vi "circle+rectangle.vi"() -> ()   [LabVIEW 2017]
uses:
  <vilib>/Simulation/Scripting/Companion Diagram/SimConfigNode/SimParams.ctl
  <vilib>/Simulation/Scripting/Companion Diagram/SimConfigNode/_simSolvers.ctl
  <vilib>/Simulation/Implementation/Shared/SIMSCR Execution Mode.ctl
  <vilib>/Simulation/Param Hierarchy/Typedefs/SIMPH Param Control Actions.ctl
  <vilib>/Simulation/Implementation/Shared/NILVSim_ParamChanged.vi
  <vilib>/Simulation/Implementation/Shared/NILVSIM_BeginStep.vi
  <vilib>/Simulation/Implementation/Shared/NILVSim_Manager.vi
  <vilib>/Utility/error.llb/Clear Errors.vi
  <vilib>/Simulation/Implementation/Shared/NILVSim_FinalizeModel.vi
  <vilib>/DAQmx/read.llb/DAQmx Read (Counter DBL 1Chan 1Samp).vi
  <vilib>/DAQmx/read.llb/DAQmx Read (Digital Bool 1Line 1Point).vi
  917b7e52-755f-4d44-bea8-9e7c9beac24e.vi
  a58f9967-76f1-4ebc-ad3d-26e75a3ca160.vi
  <vilib>/DAQmx/write.llb/DAQmx Write (Analog DBL 1Chan 1Samp).vi
  <vilib>/DAQmx/create/channels.llb/DAQmx Create Channel (AO-Voltage-Basic).vi
  <vilib>/DAQmx/create/channels.llb/DAQmx Create Channel (DI-Digital Input).vi
  <vilib>/DAQmx/create/channels.llb/DAQmx Create Channel (CI-Count Edges).vi
  <vilib>/Simulation/Implementation/Shared/SIM Unbundle Sim Info.vi
  <vilib>/Simulation/Implementation/Shared/NILVSim_Initialize.vi
  <vilib>/Simulation/Utility/Implementation/NILVSim Get Time and IsAcceptedStep.vi
  <vilib>/Simulation/Implementation/Shared/SIMSH Read Queue.vi
  <vilib>/Simulation/Implementation/Shared/NILVSim_GetModelError.vi
  <vilib>/Simulation/Implementation/Shared/SIM Bundle Sim Info.vi
  <vilib>/DAQmx/miscellaneous.llb/DAQmx Fill In Error Info.vi
  <vilib>/Simulation/Implementation/XNodeFramework/SimXNode/SimX.xnode
  <vilib>/Simulation/Model Libraries/PID/SIM PID (Parallel).vi
  <vilib>/Simulation/Model Libraries/PID/SIM PID.vi
  <vilib>/Simulation/Scripting/Companion Diagram/SimConfigNode/SimDog.xnode
  <vilib>/Simulation/Model Libraries/PID/SIM PID (Academic).vi
  <vilib>/Simulation/Implementation/Shared/NI_SIM_Implementation.lvlib
panel:
  out "Boolean 2":bool
  out "reset":bool
  in  "checking re":bool
  in  "checking enums":T1(ring)
  in  "rectangle":bool
  in  "Boolean":bool
  in  "stage rectangle":T2(ring)
  out "Step 2I":bool
  out "Step 2G":bool
  out "Step 2E":bool
  out "stay1":dbl
  out "stay":dbl
  out "calculating error x":dbl
  out "calculating error y":dbl
  in  "origin":bool
  out "Previous Y":dbl
  out "Previous X":dbl
  out "Current Y":dbl
  out "Current X":dbl
  out "previous index":dbl
  out "both/reset enter":bool
  out "reset complete":bool
  out "x circle":bool
  out "y circle":bool
  out "Point circle is drawing":dbl
  out "false":bool
  in  "Radius 2":dbl
  out "No of Points":dbl
  out "Passing Y":dbl
  out "Y array":dbl[](array[numeric])
  out "array Y length 2":dbl
  out "Passing X":dbl
  out "X array":dbl[](array[numeric])
  out "array x Length 2":dbl
  in  "stage circle":T3(ring)
  in  "check instruc":bool
  out "x entered":dbl
  out "y enetred":dbl
  out "greater -1 x":bool
  out "less 1 x":bool
  out "direction selected":dbl
  out "at 2f":bool
  out "Step 2J":bool
  out "Step 2H":bool
  out "Shape drawing steps":enum16{"corner", "1st switch", "reverse"}(ring)
  out "Step 2D":bool
  out "c":bool
  in  "height":dbl
  in  "length":dbl
  in  "part":T4(ring)=enum."a"
  in  "Has encoders been reset?":enum16{"don't reset", "reset"}(ring)
  out "x distance currently being travelled":dbl
  out "y distance currently being travelled":dbl
  out "error calced":dbl
  out "p1 dis 2":dbl
  out "p1 dis":dbl
  out "error y":dbl
  out "calc distance y":dbl
  out "calc distanc x":dbl
  out "error x":dbl
  out "reached y":bool
  out "reached x":bool
  out "Numeric":dbl
  in  "Draw rectangle":bool
  in  "Draw circle":bool
  out "In drawing mode":bool
  in  "Right-Down":bool
  in  "Left-Up":bool
  in  "Left-Down":bool
  in  "Right-Up":bool
  in  "right":bool
  in  "left":bool
  in  "motor 2":dbl(slide)=1.5 scale=-10.0..10.0
  in  "down":bool
  in  "up":bool
  in  "Y Length":dbl=30.0
  in  "X Length":dbl=30.0
  in  "Motor 2 encoder":tag="Dev1/ctr1"
  out "Pulses M2":dbl format="%.2f"
  in  "Motor 1 encoder":tag="Dev1/ctr0"
  out "Pulses M1":dbl format="%.2f"
  out "Right":bool
  out "Bottom":bool
  out "Left":bool
  out "Top":bool
  in  "Switch 4/Line 3":tag="Dev1/port0/line3"
  in  "Switch 3/Line 2":tag="Dev1/port0/line2"
  in  "Switch 2/Line 1":tag="Dev1/port0/line1"
  in  "Switch 1/Line 0":tag="Dev1/port0/line0"
  in  "Motor stop":bool
  in  "Motor 1":tag="Dev1/ao0"
  in  "max Voltage":dbl=10.0
  in  "Min Voltage":dbl=-10.0
  in  "Motor 2":tag="Dev1/ao1"
  in  "motor 1":dbl(slide)=1.5 scale=-10.0..10.0
  in  "stop":bool
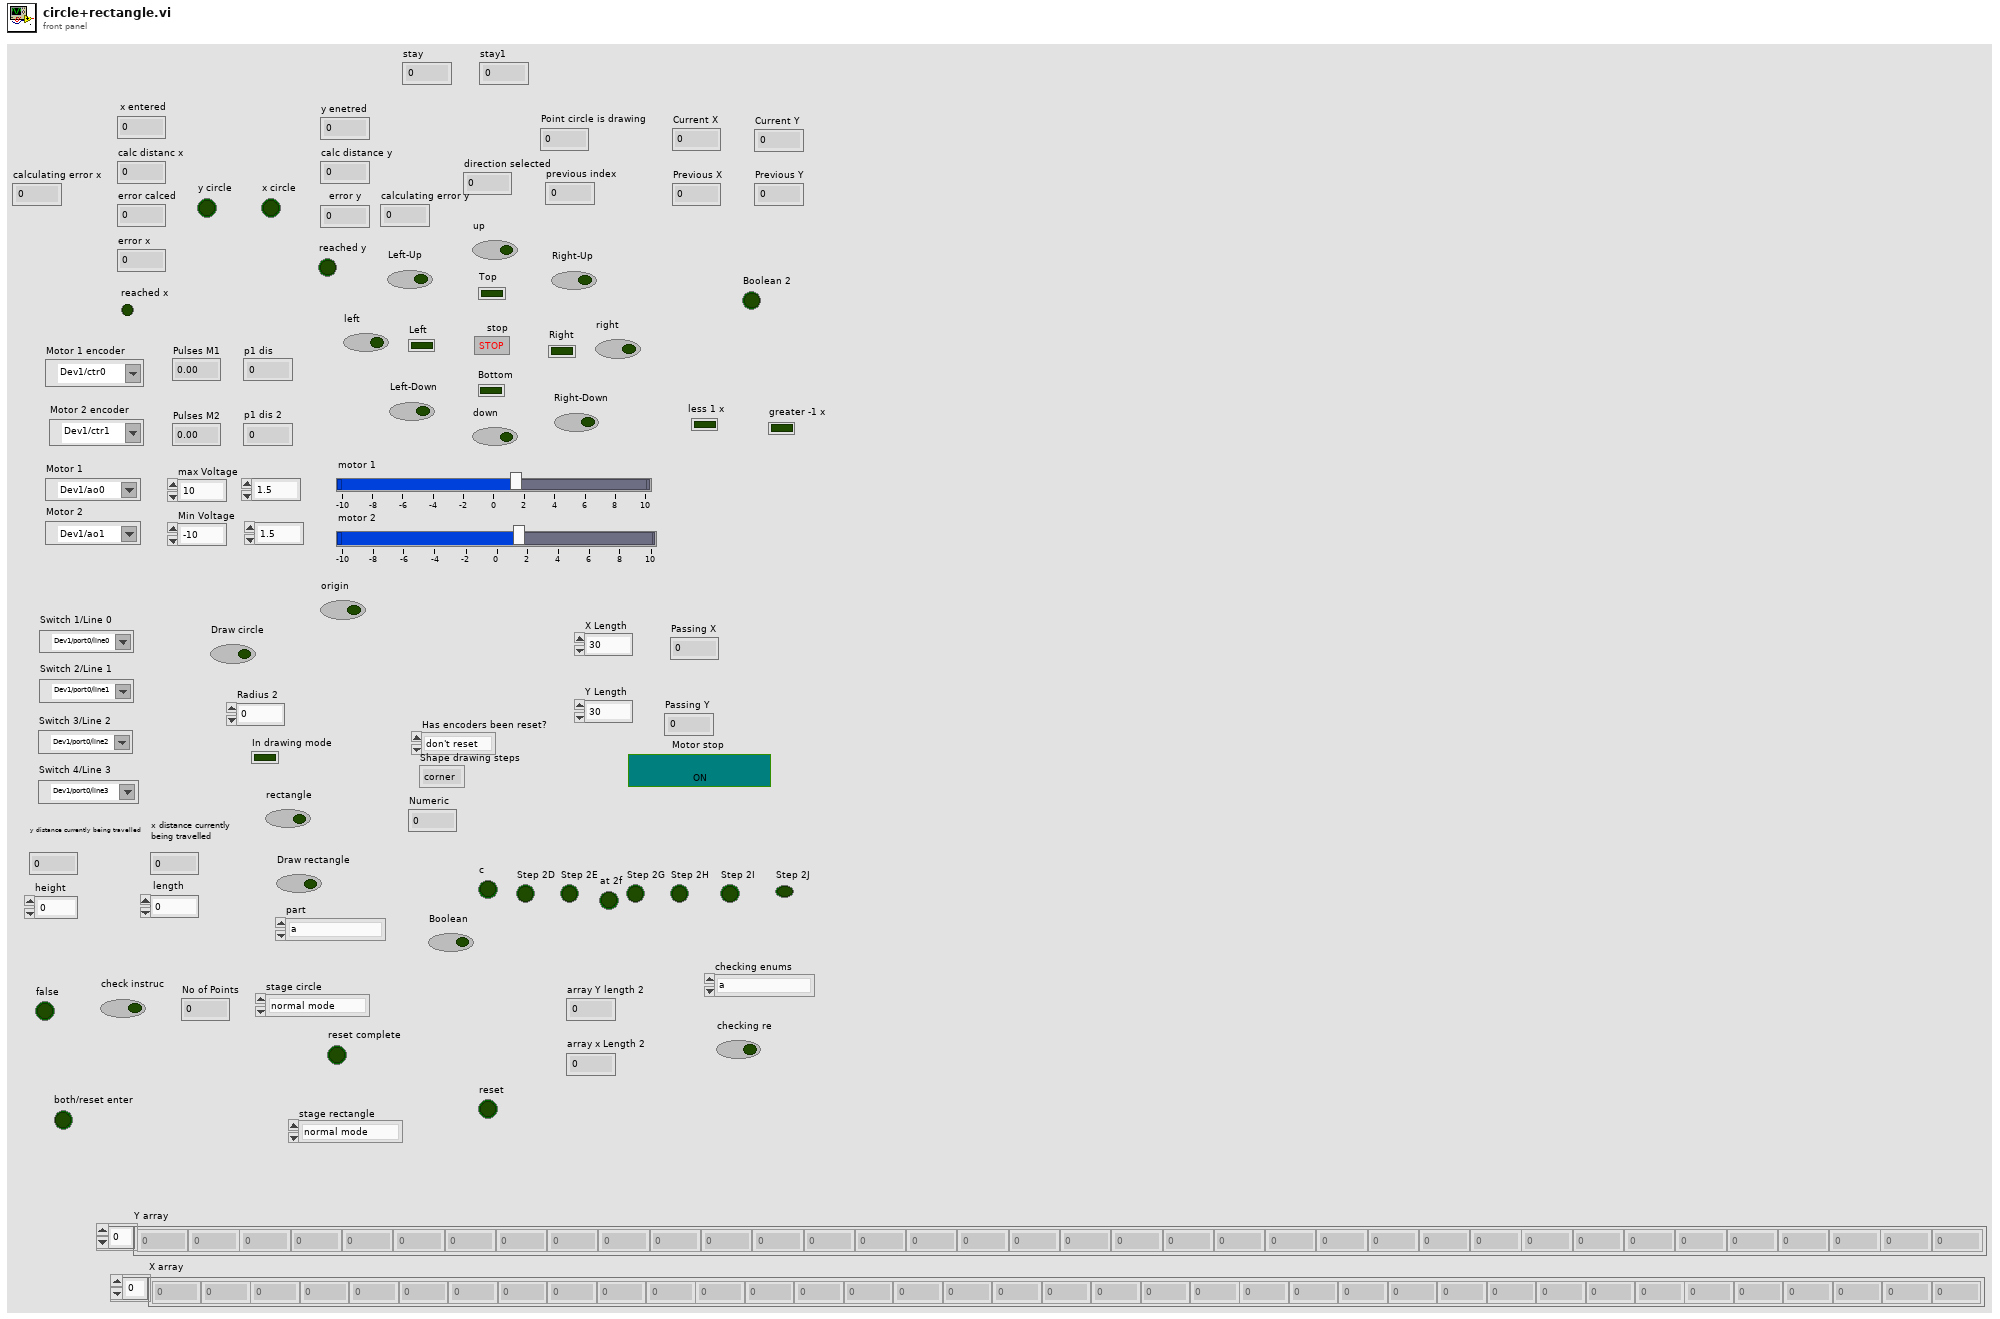
[diagram p1: front panel]
types:
  T1 = enum16{"a", "starting pt", "reset", "going right", "reset before down", "going down", "reset before left", "going left", "reset before up", "going up", "nothing"}
  T2 = enum16{"normal mode", "take to origin", "reset before start", "reset before right", "giving values right", "drawing right", "reset before down", "giving values down", "drawing down", "reset before left", "giving value left", "drawing left", "reset before up", "giving values up", "drawing up", "last step"}
  T3 = enum16{"normal mode", "take to origin", "reset before start", "create points", "draw points", "checking if draw", "reset draw counter"}
  T4 = enum16{"nothing", "j", "i", "h", "g", "f", "e", "d", "c", "b", "a"}
  T5 = enum16{"a", "starting pt", "reset", "going right", "reset before down", "going down", "reset before left", "going left", "reset before up", "going up"}
  T6 = enum16{"Simulate to Completion", "Single Time-Step Simulation (Fixed Step Only)"}
  T7 = typedef "SIMSCR Execution Mode.ctl" = enum16{"Simulate to Completion", "Single Time-Step Simulation (Fixed Step Only)"}
  T8 = typedef "SIMPH Param Control Actions.ctl" = enum16{"get params", "set params"}
  T9 = cluster{"SIMSH Sim Time":dbl, "SIM PID Derivative Gain.vi":cluster{"output":dbl}, "SIM PID Derivative Gain.vi - SIMSH":cluster{"SIMSH Sim Time":dbl, "t 3":dbl, "Select 2":cluster{"s? t:f":dbl}, "Equal?":cluster{"x = y?":bool}, "Or":cluster{"x .or. y?":bool}, "Equal To 0?":cluster{"x = 0?":bool}}, "High Frequency [s] (Tf)":dbl, "Gain":cluster{"output":dbl}, "Summation":cluster{"Result":dbl}, "Integral Gain - series.vi":cluster{"output":dbl}, "Integral Gain - series.vi - SIMSH":cluster{"SIMSH Sim Time":dbl, "Select 2":cluster{"s? t:f":dbl}, "integral in gain?":bool, "Integrator":cluster{"output y(t)":dbl}, "Gain 2":cluster{"output":dbl}, "Select":cluster{"s? t:f":dbl}, "Equal To 0?":cluster{"x = 0?":bool}, "Reciprocal":cluster{"1/x":dbl}}}
  T10 = typedef "SimParams.ctl" = cluster{"Initial Time (s)":dbl, "Final Time (s)":dbl, "Step Size (s)":dbl, "ODE Solver":T11, "Minimum Step Size (s)":dbl, "Maximum Step Size (s)":dbl, "Relative Tolerance":dbl, "Absolute Tolerance":dbl, "Software Timing":bool, "Initial Step Size (s)":dbl, "Automatic Fixed Step Size?":bool, "Automatic Discrete Step Size?":bool, "Discrete Step Size (s)":dbl, "Calculate using Time Step":bool, "Solver Wired?":bool, "Prev.Frm.Expected End":u64, "Prev.Frm.Actual End":u64, "Prev.Frm.Finished Late?":bool, "Prev.Iter.Expected End":u64, "Prev.Iter.Actual End":u64, "Prev.Iter.Finished Late?":bool, "Expected Iteration Start":u64, "Actual Iteration Start":u64, "Expected Frame Start":u64, "Actual Frame Start":u64, "Source Name":string, "Name":string, "Period":i64, "Deadline":i64, "Offset":i64, "Start":i64, "Priority":i32, "Timeout":i32, "Processor":i32, "Mode":enum32{"No Change", "Process missed periods, maintain original phase", "Discard missed periods, maintain original phase", "Process missed periods, ignore original phase", "Discard missed periods, ignore original phase"}, "Wakeup reason":enum32{"Normal", "Aborted", "Asynchronous wakeup", "Timing source error", "Timed loop error", "Timeout"}, "Error":errorcluster, "Source Type":string, "Secondary Source Type":string, "Global End Time":u64, "Global Start Time":u64, "Full Solver Reset":bool, "Execution Mode":T7, "Nan/Inf Check":bool, "Custom Solver Library":string, "Solver Is Variable":bool, "custom solver name":string, "Signal Collection Decimation":u32}
  T11 = typedef "_simSolvers.ctl" = enum16{"Runge-Kutta 1 (Euler)", "Runge-Kutta 2", "Runge-Kutta 3", "Runge-Kutta 4", "Runge-Kutta 23 (variable)", "Runge-Kutta 45 (variable)", "BDF (variable)", "Adams-Moulton (variable)", "Rosenbrock (variable)", "Discrete States Only", "SDIRK 4 (variable)", "Radau 5 (variable)", "Radau 9 (variable)", "Radau 13 (variable)", "Radau [Variable Order] (variable)", "Gear's Method (variable)", "Linearizer", "State Query", "Trim Eval", "Custom Solver"}
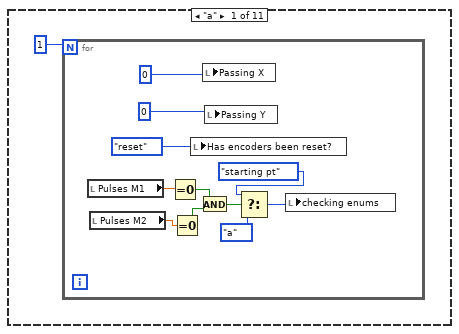
[diagram p3: hidden frame]
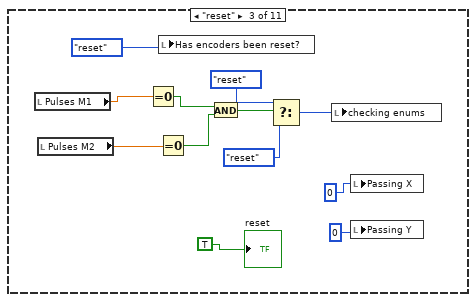
[diagram p4: hidden frame]
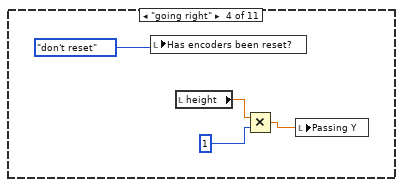
[diagram p5: hidden frame]
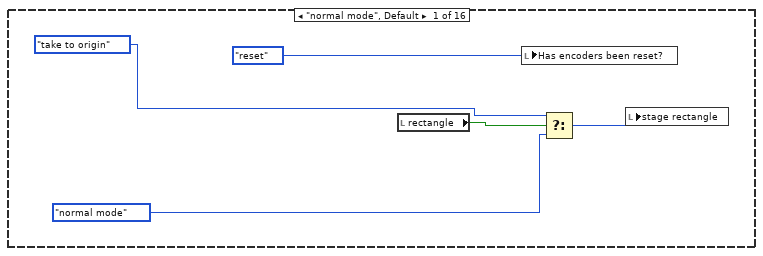
[diagram p14: hidden frame]
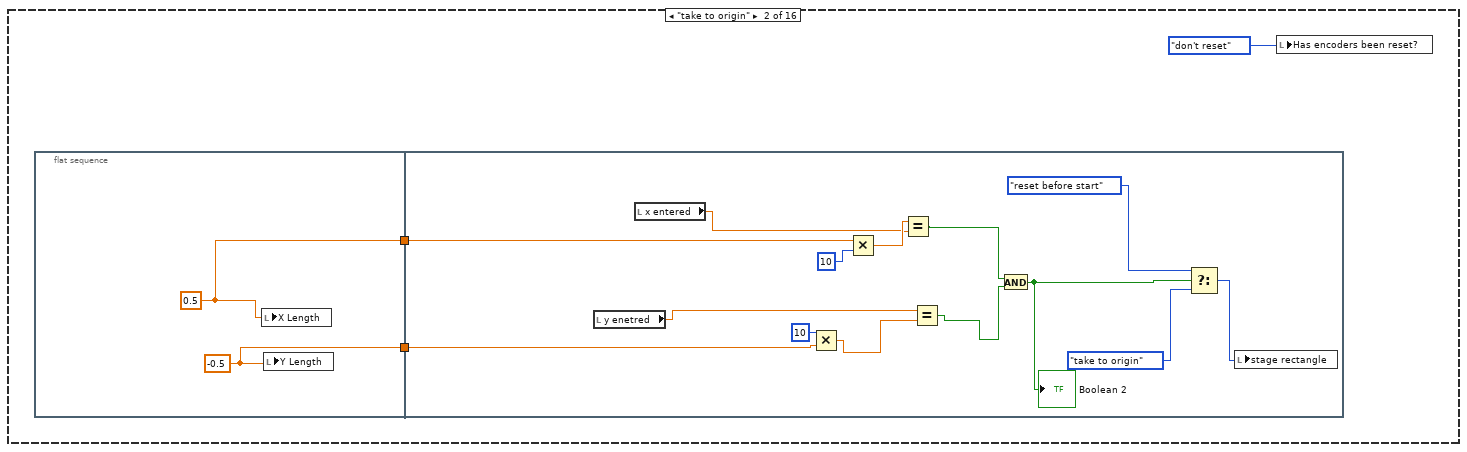
[diagram p15: hidden frame]
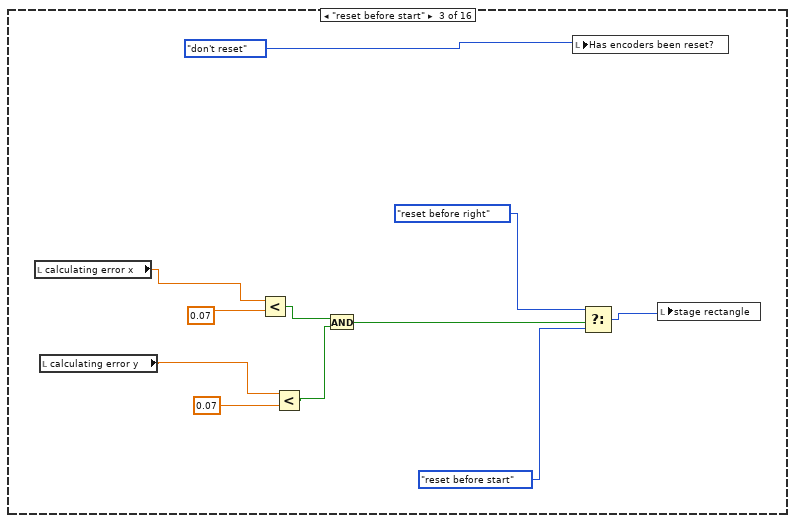
[diagram p16: hidden frame]
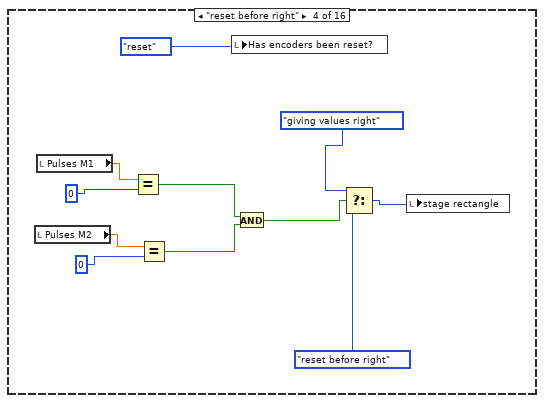
[diagram p17: hidden frame]
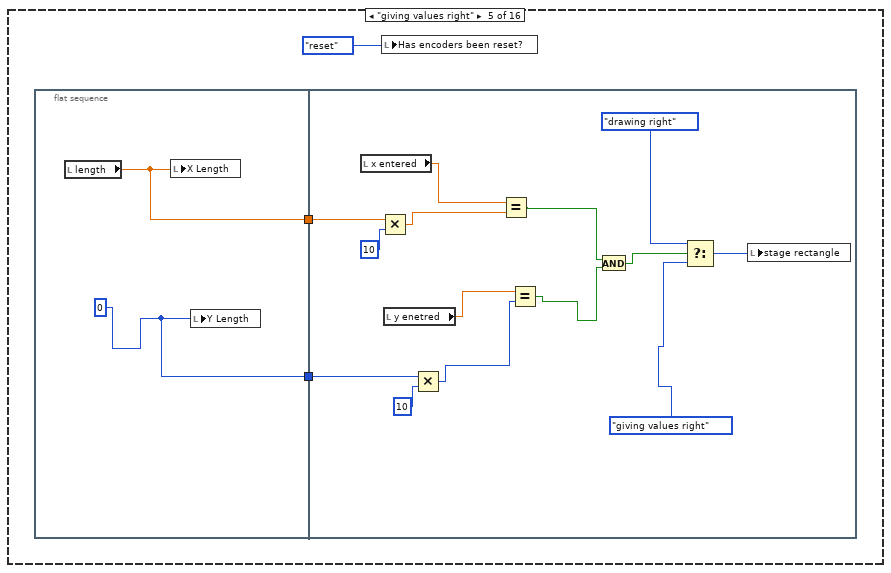
[diagram p18: hidden frame]
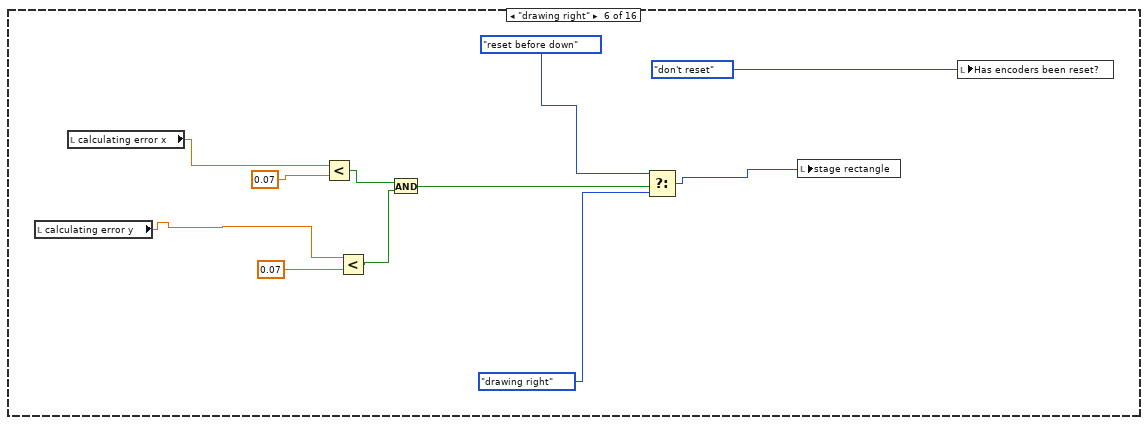
[diagram p19: hidden frame]
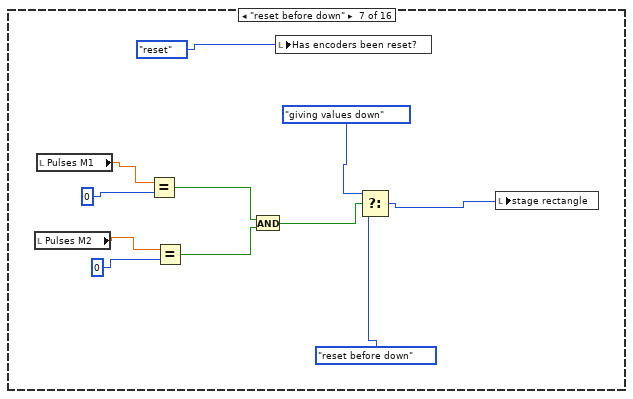
[diagram p20: hidden frame]
diagram:
  n1 = call-poly <vilib>:"DAQmx Create Virtual Channel.vi"("lines"="Switch 1/Line 0") -> ("task out"=w36:refnum<k21>, "error out"=w32:errorcluster)  [unwired: 13 in]
  n2 = call-poly <vilib>:"DAQmx Create Virtual Channel.vi"("lines"="Switch 2/Line 1") -> ("task out"=w35:refnum<k21>, "error out"=w31:errorcluster)  [unwired: 13 in]
  n3 = call-poly <vilib>:"DAQmx Create Virtual Channel.vi"("lines"="Switch 3/Line 2") -> ("task out"=w34:refnum<k21>, "error out"=w30:errorcluster)  [unwired: 13 in]
  n4 = call-poly <vilib>:"DAQmx Create Virtual Channel.vi"("lines"="Switch 4/Line 3") -> ("task out"=w33:refnum<k21>, "error out"=w29:errorcluster)  [unwired: 13 in]
  n5 = call-poly <vilib>:"DAQmx Create Virtual Channel.vi"("maximum value"="max Voltage", "minimum value"="Min Voltage", "physical channels"="Motor 1") -> ("task out"=w46:refnum<k21>, "error out"=w42:errorcluster)  [unwired: 11 in]
  n6 = call <vilib>:"DAQmx Start Task.vi"("task/channels in"=w36, "error in"=w32) -> ("task out"=w28:refnum<k21>, "error out"=w26:errorcluster)  [unwired: 12 in]
  n7 = call <vilib>:"DAQmx Start Task.vi"("task/channels in"=w35, "error in"=w31) -> ("task out"=w24:refnum<k21>, "error out"=w21:errorcluster)  [unwired: 12 in]
  n8 = call-poly <vilib>:"DAQmx Create Virtual Channel.vi"("maximum value"="max Voltage", "minimum value"="Min Voltage", "physical channels"="Motor 2") -> ("task out"=w49:refnum<k21>, "error out"=w41:errorcluster)  [unwired: 11 in]
  n9 = call-poly <vilib>:"DAQmx Create Virtual Channel.vi"("counter"="Motor 1 encoder") -> ("task out"=w7:refnum<k21>, "error out"=w2:errorcluster)  [unwired: 13 in]
  n10 = call-poly <vilib>:"DAQmx Create Virtual Channel.vi"("counter"="Motor 2 encoder") -> ("task out"=w6:refnum<k21>)  [unwired: 13 in, 1 out]
  n11 = call <vilib>:"DAQmx Start Task.vi"("task/channels in"=w34, "error in"=w30) -> ("task out"=w23:refnum<k21>, "error out"=w20:errorcluster)  [unwired: 12 in]
  n12 = call <vilib>:"DAQmx Start Task.vi"("task/channels in"=w33, "error in"=w29) -> ("task out"=w22:refnum<k21>, "error out"=w19:errorcluster)  [unwired: 12 in]
  n13 = call <vilib>:"DAQmx Start Task.vi"("task/channels in"=w7) -> ("task out"=w3:refnum<k21>)  [unwired: 13 in, 1 out]
  n14 = call <vilib>:"DAQmx Start Task.vi"("task/channels in"=w6) -> ("task out"=w1:refnum<k21>)  [unwired: 13 in, 1 out]
  n15 = while {
    tunnel: w49 -> [w240]
    tunnel: [w237] -> w48
    tunnel: w46 -> [w234]
    tunnel: [w233] -> w45
    tunnel: w42 -> [w231]
    tunnel: w41 -> [w230]
    tunnel: w28 -> [w224]
    tunnel: [w223] -> w27
    tunnel: w26 -> [w222]
    tunnel: [w221] -> w25
    tunnel: w24 -> [w220]
    tunnel: w23 -> [w219]
    tunnel: w22 -> [w218]
    tunnel: w21 -> [w217]
    tunnel: w20 -> [w216]
    tunnel: w19 -> [w215]
    tunnel: [w214] -> w18
    tunnel: [w213] -> w17
    tunnel: [w212] -> w16
    tunnel: [w211] -> w15
    tunnel: [w210] -> w14
    tunnel: [w209] -> w13
    tunnel: [w145] -> w10
    tunnel: w3 -> [w147]
    tunnel: w2 -> [w146]
    tunnel: w1 -> [w143]
    stop <- "stop" stop-if-true
    n16 = case shown="True" "check instruc" {
      frame False {
        "false" <- TRUE
      }
      frame True {
        n17 = case shown="\"reset before start\"" "stage circle" {
          frame "normal mode", Default {
            n18 = local read "check instruc"() -> (w613:bool)
            n19 = local write "Y Length"(0) -> ()
            n20 = local write "X Length"(0) -> ()
            n21 = local write "Has encoders been reset?"(enum16{"don't reset", "reset"}."reset") -> ()
            n22 = Select(t=T3."take to origin", s=w613, f=T3."normal mode") -> (s? t:f=w614:T3)
            n23 = local write "stage circle"(w614) -> ()
          }
          frame "take to origin" {
            n24 = flat-sequence {
              tunnel: [w621] -> w618
              tunnel: [w620] -> w617
              tunnel: w618 -> [w624]
              tunnel: w617 -> [w623]
              frame #0 {
                w620 = -1
                w621 = -1
                n25 = local write "X Length"(w621) -> ()
                n26 = local write "Y Length"(w620) -> ()
              }
              frame #1 {
                n27 = Multiply(x=10, y=w623) -> (x*y=w634:i32)
                n28 = local read "y enetred"() -> (w628:dbl)
                n29 = local read "x entered"() -> (w627:dbl)
                n30 = Multiply(x=10, y=w624) -> (x*y=w633:i32)
                n31 = Equal?(x=w627, y=w633) -> (x = y?=w630:bool)
                n32 = Equal?(x=w634, y=w628) -> (x = y?=w629:bool)
                n33 = And(x=w630, y=w629) -> (x .and. y?=w635:bool)
                n34 = Select(t=T3."reset before start", s=w635, f=T3."take to origin") -> (s? t:f=w622:T3)
                n35 = local write "stage circle"(w622) -> ()
              }
            }
            n36 = local write "Has encoders been reset?"(enum16{"don't reset", "reset"}."reset") -> ()
          }
          frame "reset before start" {
            n37 = local read "calculating error x"() -> (w645:dbl)
            n38 = local read "calculating error y"() -> (w643:dbl)
            n39 = Less?(x=w645, y=0.07) -> (x < y?=w641:bool)
            n40 = Less?(x=w643, y=0.07) -> (x < y?=w640:bool)
            n41 = local write "Has encoders been reset?"(enum16{"don't reset", "reset"}."don't reset") -> ()
            n42 = And(x=w641, y=w640) -> (x .and. y?=w639:bool)
            n43 = Select(t=T3."create points", s=w639, f=T3."reset before start") -> (s? t:f=w636:T3)
            n44 = local write "stage circle"(w636) -> ()
          }
          frame "create points" {
            n45 = for {
              N: 88 -> [_]
              shift-right: [w663] -> w654
              shift-left: _ -> [_]
              tunnel: [w663] -> w659 mode=indexing
              shift-right: [w662] -> w656
              shift-left: _ -> [_]
              tunnel: [w662] -> w658 mode=indexing
              i -> [w664]
              n46 = Multiply(x=2, y=3.141592653589793) -> (x*y=w667:dbl)
              n47 = Increment(x=w664) -> (x+1=w665:i32)
              n48 = Divide(x=w667, y=88) -> (x/y=w669:dbl)
              n49 = Multiply(x=w669, y=w665) -> (x*y=w666:dbl)
              n50 = Cosine(x=w666) -> (cos(x)=w672:dbl)
              n51 = Sine(x=w666) -> (sin(x)=w673:dbl)
              n52 = Multiply(x=w673, y="Radius 2") -> (x*y=w663:dbl)
              n53 = Multiply(x=w672, y="Radius 2") -> (x*y=w662:dbl)
              "No of Points" <- w664
            }
            "Passing Y" <- w654
            "Y array" <- w659
            "Passing X" <- w656
            "X array" <- w658
            n54 = local read "No of Points"() -> (w653:dbl)
            n55 = Equal?(x=w653, y=87) -> (x = y?=w650:bool)
            n56 = local write "Has encoders been reset?"(enum16{"don't reset", "reset"}."don't reset") -> ()
            n57 = Select(t=T3."draw points", s=w650, f=T3."create points") -> (s? t:f=w660:T3)
            n58 = local write "stage circle"(w660) -> ()
            n59 = Array Size(array=w659) -> (size(s)=→"array Y length 2":i32)
            n60 = Array Size(array=w658) -> (size(s)=→"array x Length 2":i32)
          }
          frame "draw points" {
            n61 = flat-sequence {
              frame #0 {
                n62 = local read "Point circle is drawing"() -> (w702:dbl)
                n63 = local read "previous index"() -> (w694:dbl)
                n64 = local read "Y array"() -> (w695:dbl[])
                n65 = local read "X array"() -> (w696:dbl[])
                n66 = Index Array(array=w695, index=w694) -> (element=→"Previous Y":dbl)
                n67 = Index Array(array=w696, index=w694) -> (element=→"Previous X":dbl)
                n68 = local read "X array"() -> (w697:dbl[])
                n69 = local read "Previous X"() -> (w684:dbl)
                n70 = local read "Current X"() -> (w689:dbl)
                n71 = local read "Y array"() -> (w698:dbl[])
                n72 = local read "Current X"() -> (w687:dbl)
                n73 = Greater Or Equal?(x=w702, y=89) -> (x >= y?=w700:bool)
                n74 = Not Equal To 0?(x=w702) -> (x != 0?=w690:bool)
                n75 = local read "Previous Y"() -> (w685:dbl)
                n76 = local read "Current Y"() -> (w686:dbl)
                n77 = Index Array(array=w697, index=w702) -> (element=→"Current X":dbl)
                n78 = Subtract(x=w687, y=w684) -> (x-y=w682:dbl)
                n79 = Select(t=w682, s=w690, f=w689) -> (s? t:f=w679:dbl)
                n80 = Select(t=T3."normal mode", s=w700, f=T3."draw points") -> (s? t:f=w699:T3)
                n81 = Index Array(array=w698, index=w702) -> (element=→"Current Y":dbl)
                n82 = Subtract(x=w686, y=w685) -> (x-y=w681:dbl)
                n83 = local read "Current Y"() -> (w688:dbl)
                n84 = local write "X Length"(w679) -> ()
                n85 = Not(x=w700) -> (.not. x?=w701:bool)
                n86 = local write "stage circle"(w699) -> ()
                n87 = Not Equal To 0?(x=w702) -> (x != 0?=w691:bool)
                n88 = Select(t=w681, s=w691, f=w688) -> (s? t:f=w680:dbl)
                n89 = local write "Y Length"(w680) -> ()
                n90 = local write "check instruc"(w701) -> ()
              }
              frame #1 {
                n91 = local write "stage circle"(T3."checking if draw") -> ()
              }
            }
            n92 = local write "Has encoders been reset?"(enum16{"don't reset", "reset"}."don't reset") -> ()
          }
          frame "checking if draw" {
            n93 = local read "calculating error x"() -> (w707:dbl)
            n94 = local read "calculating error y"() -> (w705:dbl)
            n95 = local read "Point circle is drawing"() -> (w710:dbl)
            n96 = Greater Or Equal?(x=0.07, y=w707) -> (x >= y?=w713:bool)
            "x circle" <- w713
            n97 = Greater Or Equal?(x=0.07, y=w705) -> (x >= y?=w714:bool)
            "y circle" <- w714
            n98 = And(x=w714, y=w713) -> (x .and. y?=w711:bool)
            "both/reset enter" <- w711
            n99 = Increment(x=w710) -> (x+1=w716:dbl)
            n100 = Select(t=w716, s=w711, f=w710) -> (s? t:f=→"Point circle is drawing":dbl)
            n101 = Select(t=T3."reset draw counter", s=w711, f=T3."checking if draw") -> (s? t:f=w712:T3)
            n102 = local write "stage circle"(w712) -> ()
          }
          frame "reset draw counter" {
            n103 = for {
              N: 1 -> [_]
              i -> [w721]
              n104 = local read "Point circle is drawing"() -> (w726:dbl)
              n105 = local read "Pulses M2"() -> (w731:dbl)
              n106 = local read "Pulses M1"() -> (w732:dbl)
              n107 = Equal To 0?(x=w731) -> (x = 0?=w730:bool)
              n108 = Equal To 0?(x=w732) -> (x = 0?=w728:bool)
              n109 = local read "previous index"() -> (w723:dbl)
              n110 = local write "Has encoders been reset?"(enum16{"don't reset", "reset"}."reset") -> ()
              n111 = And(x=w728, y=w730) -> (x .and. y?=w729:bool)
              n112 = Subtract(x=w726, y=1) -> (x-y=w724:dbl)
              n113 = Select(t=T3."draw points", s=w729, f=T3."reset draw counter") -> (s? t:f=w733:T3)
              n114 = Equal To 0?(x=w721) -> (x = 0?=w720:bool)
              n115 = local write "stage circle"(w733) -> ()
              n116 = Select(t=w724, s=w720, f=w723) -> (s? t:f=→"previous index":dbl)
              "reset complete" <- TRUE
            }
          }
        }
      }
    }
    n117 = case shown="True" "rectangle" {
      frame False {
      }
      frame True {
        n118 = case shown="\"giving value left\"" "stage rectangle" {
          frame "normal mode", Default {
            n119 = local read "rectangle"() -> (w288:bool)
            n120 = local write "Has encoders been reset?"(enum16{"don't reset", "reset"}."reset") -> ()
            n121 = Select(t=T2."take to origin", s=w288, f=T2."normal mode") -> (s? t:f=w286:T2)
            n122 = local write "stage rectangle"(w286) -> ()
          }
          frame "take to origin" {
            n123 = flat-sequence {
              tunnel: [w293] -> w290
              tunnel: [w292] -> w289
              tunnel: w290 -> [w303]
              tunnel: w289 -> [w302]
              frame #0 {
                w293 = -0.5
                w292 = 0.5
                n124 = local write "X Length"(w292) -> ()
                n125 = local write "Y Length"(w293) -> ()
              }
              frame #1 {
                n126 = local read "y enetred"() -> (w297:dbl)
                n127 = local read "x entered"() -> (w298:dbl)
                n128 = Multiply(x=10, y=w303) -> (x*y=w305:dbl)
                n129 = Multiply(x=w302, y=10) -> (x*y=w301:dbl)
                n130 = Equal?(x=w301, y=w298) -> (x = y?=w300:bool)
                n131 = Equal?(x=w297, y=w305) -> (x = y?=w299:bool)
                n132 = And(x=w300, y=w299) -> (x .and. y?=w307:bool)
                "Boolean 2" <- w307
                n133 = Select(t=T2."reset before start", s=w307, f=T2."take to origin") -> (s? t:f=w296:T2)
                n134 = local write "stage rectangle"(w296) -> ()
              }
            }
            n135 = local write "Has encoders been reset?"(enum16{"don't reset", "reset"}."don't reset") -> ()
          }
          frame "reset before start" {
            n136 = local read "calculating error x"() -> (w312:dbl)
            n137 = local read "calculating error y"() -> (w311:dbl)
            n138 = Less?(x=w312, y=0.07) -> (x < y?=w313:bool)
            n139 = Less?(x=w311, y=0.07) -> (x < y?=w315:bool)
            n140 = And(x=w313, y=w315) -> (x .and. y?=w310:bool)
            n141 = local write "Has encoders been reset?"(enum16{"don't reset", "reset"}."don't reset") -> ()
            n142 = Select(t=T2."reset before right", s=w310, f=T2."reset before start") -> (s? t:f=w317:T2)
            n143 = local write "stage rectangle"(w317) -> ()
          }
          frame "reset before right" {
            n144 = local read "Pulses M2"() -> (w328:dbl)
            n145 = local read "Pulses M1"() -> (w329:dbl)
            n146 = Equal?(x=w329, y=0) -> (x = y?=w327:bool)
            n147 = Equal?(x=w328, y=0) -> (x = y?=w326:bool)
            n148 = local write "Has encoders been reset?"(enum16{"don't reset", "reset"}."reset") -> ()
            n149 = And(x=w327, y=w326) -> (x .and. y?=w325:bool)
            n150 = Select(t=T2."giving values right", s=w325, f=T2."reset before right") -> (s? t:f=w324:T2)
            n151 = local write "stage rectangle"(w324) -> ()
          }
          frame "giving values right" {
            n152 = flat-sequence {
              tunnel: [w333] -> w332
              tunnel: [w334] -> w331
              tunnel: w332 -> [w344]
              tunnel: w331 -> [w343]
              frame #0 {
                w333 = 0
                n153 = local read "length"() -> (w334:dbl)
                n154 = local write "X Length"(w334) -> ()
                n155 = local write "Y Length"(w333) -> ()
              }
              frame #1 {
                n156 = local read "x entered"() -> (w341:dbl)
                n157 = Multiply(x=w343, y=10) -> (x*y=w342:dbl)
                n158 = local read "y enetred"() -> (w339:dbl)
                n159 = Multiply(x=w344, y=10) -> (x*y=w340:i32)
                n160 = Equal?(x=w341, y=w342) -> (x = y?=w346:bool)
                n161 = Equal?(x=w339, y=w340) -> (x = y?=w345:bool)
                n162 = And(x=w346, y=w345) -> (x .and. y?=w337:bool)
                n163 = Select(t=T2."drawing right", s=w337, f=T2."giving values right") -> (s? t:f=w338:T2)
                n164 = local write "stage rectangle"(w338) -> ()
              }
            }
            n165 = local write "Has encoders been reset?"(enum16{"don't reset", "reset"}."reset") -> ()
          }
          frame "drawing right" {
            n166 = local read "calculating error y"() -> (w356:dbl)
            n167 = local read "calculating error x"() -> (w355:dbl)
            n168 = Less?(x=w355, y=0.07) -> (x < y?=w358:bool)
            n169 = Less?(x=w356, y=0.07) -> (x < y?=w359:bool)
            n170 = And(x=w358, y=w359) -> (x .and. y?=w357:bool)
            n171 = Select(t=T2."reset before down", s=w357, f=T2."drawing right") -> (s? t:f=w354:T2)
            n172 = local write "stage rectangle"(w354) -> ()
            n173 = local write "Has encoders been reset?"(enum16{"don't reset", "reset"}."don't reset") -> ()
          }
          frame "reset before down" {
            n174 = local read "Pulses M2"() -> (w364:dbl)
            n175 = local read "Pulses M1"() -> (w365:dbl)
            n176 = Equal?(x=w365, y=0) -> (x = y?=w370:bool)
            n177 = Equal?(x=w364, y=0) -> (x = y?=w369:bool)
            n178 = And(x=w370, y=w369) -> (x .and. y?=w368:bool)
            n179 = local write "Has encoders been reset?"(enum16{"don't reset", "reset"}."reset") -> ()
            n180 = Select(t=T2."giving values down", s=w368, f=T2."reset before down") -> (s? t:f=w361:T2)
            n181 = local write "stage rectangle"(w361) -> ()
          }
          frame "giving values down" {
            n182 = flat-sequence {
              tunnel: [w377] -> w373
              tunnel: [w374] -> w372
              tunnel: w373 -> [w382]
              tunnel: w372 -> [w381]
              frame #0 {
                w377 = 0
                n183 = local read "height"() -> (w376:dbl)
                n184 = Multiply(x=w376, y=-1) -> (x*y=w374:dbl)
                n185 = local write "X Length"(w377) -> ()
                n186 = local write "Y Length"(w374) -> ()
              }
              frame #1 {
                n187 = local read "y enetred"() -> (w383:dbl)
                n188 = local read "x entered"() -> (w384:dbl)
                n189 = Multiply(x=w382, y=10) -> (x*y=w390:i32)
                n190 = Multiply(x=w381, y=10) -> (x*y=w388:dbl)
                n191 = Equal?(x=w384, y=w390) -> (x = y?=w385:bool)
                n192 = Equal?(x=w383, y=w388) -> (x = y?=w386:bool)
                n193 = And(x=w385, y=w386) -> (x .and. y?=w387:bool)
                n194 = Select(t=T2."drawing down", s=w387, f=T2."giving values down") -> (s? t:f=w378:T2)
                n195 = local write "stage rectangle"(w378) -> ()
              }
            }
            n196 = local write "Has encoders been reset?"(enum16{"don't reset", "reset"}."reset") -> ()
          }
          frame "drawing down" {
            n197 = local read "calculating error y"() -> (w397:dbl)
            n198 = local read "calculating error x"() -> (w396:dbl)
            n199 = Less?(x=w396, y=0.07) -> (x < y?=w401:bool)
            n200 = Less?(x=w397, y=0.07) -> (x < y?=w402:bool)
            n201 = And(x=w401, y=w402) -> (x .and. y?=w400:bool)
            n202 = Select(t=T2."reset before left", s=w400, f=T2."drawing down") -> (s? t:f=w393:T2)
            n203 = local write "Has encoders been reset?"(enum16{"don't reset", "reset"}."don't reset") -> ()
            n204 = local write "stage rectangle"(w393) -> ()
          }
          frame "reset before left" {
            n205 = local read "Pulses M1"() -> (w409:dbl)
            n206 = local read "Pulses M2"() -> (w408:dbl)
            n207 = Equal?(x=w409, y=0) -> (x = y?=w413:bool)
            n208 = Equal?(x=w408, y=0) -> (x = y?=w412:bool)
            n209 = And(x=w413, y=w412) -> (x .and. y?=w407:bool)
            n210 = Select(t=T2."giving value left", s=w407, f=T2."reset before left") -> (s? t:f=w404:T2)
            n211 = local write "stage rectangle"(w404) -> ()
            n212 = local write "Has encoders been reset?"(enum16{"don't reset", "reset"}."reset") -> ()
          }
          frame "giving value left" {
            n213 = flat-sequence {
              tunnel: [w420] -> w416
              tunnel: [w417] -> w415
              tunnel: w416 -> [w430]
              tunnel: w415 -> [w429]
              frame #0 {
                w420 = 0
                n214 = local read "length"() -> (w418:dbl)
                n215 = Multiply(x=w418, y=-1) -> (x*y=w417:dbl)
                n216 = local write "X Length"(w417) -> ()
                n217 = local write "Y Length"(w420) -> ()
              }
              frame #1 {
                n218 = local read "x entered"() -> (w428:dbl)
                n219 = local read "y enetred"() -> (w427:dbl)
                n220 = Multiply(x=w429, y=10) -> (x*y=w433:dbl)
                n221 = Multiply(x=w430, y=10) -> (x*y=w431:i32)
                n222 = Equal?(x=w428, y=w433) -> (x = y?=w425:bool)
                n223 = Equal?(x=w427, y=w431) -> (x = y?=w424:bool)
                n224 = And(x=w425, y=w424) -> (x .and. y?=w426:bool)
                n225 = Select(t=T2."drawing left", s=w426, f=T2."giving value left") -> (s? t:f=w421:T2)
                n226 = local write "stage rectangle"(w421) -> ()
              }
            }
            n227 = local write "Has encoders been reset?"(enum16{"don't reset", "reset"}."reset") -> ()
          }
          frame "drawing left" {
            n228 = local read "calculating error x"() -> (w439:dbl)
            n229 = local read "calculating error y"() -> (w440:dbl)
            n230 = Less?(x=w439, y=0.07) -> (x < y?=w444:bool)
            n231 = Less?(x=w440, y=0.07) -> (x < y?=w445:bool)
            n232 = And(x=w444, y=w445) -> (x .and. y?=w443:bool)
            n233 = Select(t=T2."reset before up", s=w443, f=T2."drawing left") -> (s? t:f=w436:T2)
            n234 = local write "Has encoders been reset?"(enum16{"don't reset", "reset"}."don't reset") -> ()
            n235 = local write "stage rectangle"(w436) -> ()
          }
          frame "reset before up" {
            n236 = local read "Pulses M1"() -> (w451:dbl)
            n237 = local read "Pulses M2"() -> (w450:dbl)
            n238 = Equal?(x=w451, y=0) -> (x = y?=w456:bool)
            n239 = Equal?(x=w450, y=0) -> (x = y?=w455:bool)
            n240 = And(x=w456, y=w455) -> (x .and. y?=w452:bool)
            n241 = Select(t=T2."giving values up", s=w452, f=T2."reset before up") -> (s? t:f=w447:T2)
            n242 = local write "Has encoders been reset?"(enum16{"don't reset", "reset"}."reset") -> ()
            n243 = local write "stage rectangle"(w447) -> ()
          }
          frame "giving values up" {
            n244 = flat-sequence {
              tunnel: [w461] -> w459
              tunnel: [w460] -> w458
              tunnel: w459 -> [w471]
              tunnel: w458 -> [w470]
              frame #0 {
                w460 = 0
                n245 = local read "height"() -> (w461:dbl)
                n246 = local write "X Length"(w460) -> ()
                n247 = local write "Y Length"(w461) -> ()
              }
              frame #1 {
                n248 = local read "x entered"() -> (w473:dbl)
                n249 = local read "y enetred"() -> (w472:dbl)
                n250 = Multiply(x=w470, y=10) -> (x*y=w475:i32)
                n251 = Multiply(x=w471, y=10) -> (x*y=w474:dbl)
                n252 = Equal?(x=w473, y=w475) -> (x = y?=w468:bool)
                n253 = Equal?(x=w472, y=w474) -> (x = y?=w467:bool)
                n254 = And(x=w468, y=w467) -> (x .and. y?=w469:bool)
                n255 = Select(t=T2."drawing up", s=w469, f=T2."giving values up") -> (s? t:f=w464:T2)
                n256 = local write "stage rectangle"(w464) -> ()
              }
            }
            n257 = local write "Has encoders been reset?"(enum16{"don't reset", "reset"}."reset") -> ()
          }
          frame "drawing up" {
            n258 = local read "calculating error x"() -> (w481:dbl)
            n259 = local read "calculating error y"() -> (w480:dbl)
            n260 = Less?(x=w481, y=0.07) -> (x < y?=w485:bool)
            n261 = Less?(x=w480, y=0.07) -> (x < y?=w486:bool)
            n262 = And(x=w485, y=w486) -> (x .and. y?=w484:bool)
            n263 = Select(t=T2."last step", s=w484, f=T2."drawing up") -> (s? t:f=w477:T2)
            n264 = local write "Has encoders been reset?"(enum16{"don't reset", "reset"}."don't reset") -> ()
            n265 = local write "stage rectangle"(w477) -> ()
          }
          frame "last step" {
            n266 = local write "X Length"(0) -> ()
            n267 = local write "Y Length"(0) -> ()
            n268 = local write "Has encoders been reset?"(enum16{"don't reset", "reset"}."reset") -> ()
          }
        }
      }
    }
    n269 = case shown="True" "checking re" {
      frame False {
      }
      frame True {
        n270 = case shown="\"starting pt\"" "checking enums" {
          frame "a" {
            n271 = for {
              N: 1 -> [_]
              n272 = local read "Pulses M1"() -> (w250:dbl)
              n273 = local read "Pulses M2"() -> (w249:dbl)
              n274 = Equal To 0?(x=w250) -> (x = 0?=w248:bool)
              n275 = Equal To 0?(x=w249) -> (x = 0?=w243:bool)
              n276 = local write "Has encoders been reset?"(enum16{"don't reset", "reset"}."reset") -> ()
              n277 = And(x=w248, y=w243) -> (x .and. y?=w247:bool)
              n278 = local write "Passing X"(0) -> ()
              n279 = local write "Passing Y"(0) -> ()
              n280 = Select(t=T5."starting pt", s=w247, f=T5."a") -> (s? t:f=w244:T5)
              n281 = local write "checking enums"(w244) -> ()
            }
          }
          frame "starting pt" {
            n282 = flat-sequence {
              frame #0 {
                n283 = local write "Passing Y"(10) -> ()
                n284 = local write "Passing X"(-6) -> ()
              }
            }
            n285 = local read "calculating error x"() -> (w263:dbl)
            n286 = local read "calculating error y"() -> (w261:dbl)
            n287 = local write "Has encoders been reset?"(enum16{"don't reset", "reset"}."don't reset") -> ()
            n288 = Less?(x=w263, y=0.07) -> (x < y?=w258:bool)
            n289 = Less?(x=w261, y=0.07) -> (x < y?=w259:bool)
            n290 = And(x=w258, y=w259) -> (x .and. y?=w257:bool)
            n291 = Select(t=T5."reset", s=w257, f=T5."starting pt") -> (s? t:f=w254:T5)
            n292 = local write "checking enums"(w254) -> ()
          }
          frame "reset" {
            (unwired) 0
            n293 = local read "Pulses M1"() -> (w277:dbl)
            n294 = local read "Pulses M2"() -> (w276:dbl)
            n295 = Equal To 0?(x=w277) -> (x = 0?=w274:bool)
            n296 = Equal To 0?(x=w276) -> (x = 0?=w275:bool)
            n297 = local write "Has encoders been reset?"(enum16{"don't reset", "reset"}."reset") -> ()
            n298 = And(x=w274, y=w275) -> (x .and. y?=w273:bool)
            n299 = Select(t=T5."reset", s=w273, f=T5."reset") -> (s? t:f=w270:T5)
            n300 = local write "checking enums"(w270) -> ()
            n301 = local write "Passing X"(0) -> ()
            n302 = local write "Passing Y"(0) -> ()
            "reset" <- TRUE
          }
          frame "going right" {
            n303 = local write "Has encoders been reset?"(enum16{"don't reset", "reset"}."don't reset") -> ()
            n304 = local read "height"() -> (w280:dbl)
            n305 = Multiply(x=w280, y=1) -> (x*y=w281:dbl)
            n306 = local write "Passing Y"(w281) -> ()
          }
          frame "reset before down" {
          }
          frame "going down" {
          }
          frame "reset before left" {
          }
          frame "going left" {
          }
          frame "reset before up" {
          }
          frame "going up" {
          }
          frame "nothing" {
          }
        }
      }
    }
    n307 = case shown="True" "Boolean" {
      frame False {
      }
      frame True {
        n308 = case shown="\"d\"" "part" {
          frame "a" {
            n309 = for {
              N: 1 -> [_]
              n310 = local read "Pulses M1"() -> (w498:dbl)
              n311 = local read "Pulses M2"() -> (w497:dbl)
              n312 = Equal To 0?(x=w497) -> (x = 0?=w500:bool)
              n313 = Equal To 0?(x=w498) -> (x = 0?=w499:bool)
              n314 = local write "Has encoders been reset?"(enum16{"don't reset", "reset"}."reset") -> ()
              n315 = And(x=w499, y=w500) -> (x .and. y?=w492:bool)
              n316 = local write "Passing X"(0) -> ()
              n317 = local write "Passing Y"(0) -> ()
              n318 = Select(t=T4."b", s=w492, f=T4."a") -> (s? t:f=w495:T4)
              n319 = local write "part"(w495) -> ()
            }
          }
          frame "b" {
            n320 = local read "calculating error x"() -> (w511:dbl)
            n321 = local read "calculating error y"() -> (w508:dbl)
            n322 = Greater?(x=w511, y=0.07) -> (0:w510:bool)
            n323 = Greater?(x=w508, y=0.07) -> (0:w506:bool)
            n324 = local write "Has encoders been reset?"(enum16{"don't reset", "reset"}."don't reset") -> ()
            n325 = local write "Passing Y"(1) -> ()
            n326 = local write "Passing X"(1) -> ()
            n327 = And(x=w510, y=w506) -> (x .and. y?=w513:bool)
            n328 = Select(t=T4."c", s=w513, f=T4."b") -> (s? t:f=w514:T4)
            n329 = local write "part"(w514) -> ()
          }
          frame "c" {
            n330 = for {
              N: 0 -> [_]
              n331 = local read "Pulses M2"() -> (w527:dbl)
              n332 = local read "Pulses M1"() -> (w526:dbl)
              n333 = Equal To 0?(x=w527) -> (x = 0?=w525:bool)
              n334 = Equal To 0?(x=w526) -> (x = 0?=w524:bool)
              n335 = local write "Has encoders been reset?"(enum16{"don't reset", "reset"}."reset") -> ()
              n336 = And(x=w525, y=w524) -> (x .and. y?=w523:bool)
              n337 = Select(t=T4."d", s=w523, f=T4."c") -> (s? t:f=w520:T4)
              n338 = local write "part"(w520) -> ()
            }
            n339 = local write "Passing Y"(0) -> ()
            n340 = local write "Passing X"(0) -> ()
            "c" <- TRUE
          }
          frame "d" {
            n341 = local read "calculating error y"() -> (w530:dbl)
            n342 = Multiply(x="height", y=-1) -> (x*y=w531:dbl)
            n343 = local write "Has encoders been reset?"(enum16{"don't reset", "reset"}."don't reset") -> ()
            n344 = local write "Passing X"(0) -> ()
            n345 = local write "Passing Y"(w531) -> ()
            n346 = Equal To 0?(x=w530) -> (x = 0?=w529:bool)
            "Step 2D" <- w529
            n347 = Select(t=T4."e", s=w529, f=T4."d") -> (s? t:f=w538:T4)
            n348 = local write "part"(w538) -> ()
          }
          frame "e" {
            n349 = for {
              N: 1 -> [_]
              n350 = local read "Pulses M1"() -> (w545:dbl)
              n351 = local read "Pulses M2"() -> (w544:dbl)
              n352 = Equal To 0?(x=w544) -> (x = 0?=w550:bool)
              n353 = Equal To 0?(x=w545) -> (x = 0?=w551:bool)
              n354 = local write "Has encoders been reset?"(enum16{"don't reset", "reset"}."reset") -> ()
              n355 = And(x=w551, y=w550) -> (x .and. y?=w549:bool)
              n356 = Select(t=T4."f", s=w549, f=T4."e") -> (s? t:f=w543:T4)
              n357 = local write "part"(w543) -> ()
              "Step 2E" <- TRUE
            }
            n358 = local write "Passing X"(0) -> ()
            n359 = local write "Passing Y"(0) -> ()
          }
          frame "f" {
            n360 = local read "calculating error x"() -> (w553:dbl)
            n361 = Equal To 0?(x=w553) -> (x = 0?=w552:bool)
            "at 2f" <- w552
            n362 = local write "Passing Y"(0) -> ()
            n363 = local write "Passing X"("length") -> ()
            n364 = local write "Has encoders been reset?"(enum16{"don't reset", "reset"}."don't reset") -> ()
            n365 = Select(t=T4."g", s=w552, f=T4."f") -> (s? t:f=w557:T4)
            n366 = local write "part"(w557) -> ()
          }
          frame "g" {
            n367 = for {
              N: 1 -> [_]
              n368 = local read "Pulses M1"() -> (w565:dbl)
              n369 = local read "Pulses M2"() -> (w564:dbl)
              n370 = Equal To 0?(x=w565) -> (x = 0?=w572:bool)
              n371 = Equal To 0?(x=w564) -> (x = 0?=w571:bool)
              n372 = local write "Has encoders been reset?"(enum16{"don't reset", "reset"}."reset") -> ()
              n373 = And(x=w572, y=w571) -> (x .and. y?=w570:bool)
              n374 = Select(t=T4."h", s=w570, f=T4."g") -> (s? t:f=w567:T4)
              n375 = local write "part"(w567) -> ()
            }
            n376 = local write "Passing X"(0) -> ()
            n377 = local write "Passing Y"(0) -> ()
            "Step 2G" <- TRUE
          }
          frame "h" {
            n378 = local read "height"() -> (w575:dbl)
            n379 = local read "calculating error y"() -> (w573:dbl)
            n380 = local write "Passing X"(0) -> ()
            n381 = local write "Passing Y"(w575) -> ()
            n382 = local write "Has encoders been reset?"(enum16{"don't reset", "reset"}."don't reset") -> ()
            n383 = Equal To 0?(x=w573) -> (x = 0?=w574:bool)
            n384 = Select(t=T4."i", s=w574, f=T4."h") -> (s? t:f=w578:T4)
            n385 = local write "part"(w578) -> ()
            "Step 2H" <- TRUE
          }
          frame "i" {
            n386 = for {
              N: 1 -> [_]
              n387 = local read "Pulses M1"() -> (w588:dbl)
              n388 = local read "Pulses M2"() -> (w587:dbl)
              n389 = Equal To 0?(x=w587) -> (x = 0?=w593:bool)
              n390 = Equal To 0?(x=w588) -> (x = 0?=w594:bool)
              n391 = And(x=w594, y=w593) -> (x .and. y?=w592:bool)
              n392 = local write "Has encoders been reset?"(enum16{"don't reset", "reset"}."reset") -> ()
              n393 = Select(t=T4."j", s=w592, f=T4."i") -> (s? t:f=w586:T4)
              n394 = local write "part"(w586) -> ()
            }
            n395 = local write "Passing Y"(0) -> ()
            n396 = local write "Passing X"(0) -> ()
            "Step 2I" <- TRUE
          }
          frame "j" {
            n397 = local read "calculating error x"() -> (w599:dbl)
            n398 = local read "length"() -> (w596:dbl)
            n399 = Equal To 0?(x=w599) -> (x = 0?=w598:bool)
            n400 = Multiply(x=w596, y=-1) -> (x*y=w595:dbl)
            n401 = local write "Has encoders been reset?"(enum16{"don't reset", "reset"}."don't reset") -> ()
            n402 = local write "Passing Y"(0) -> ()
            n403 = local write "Passing X"(w595) -> ()
            n404 = Select(t=T4."nothing", s=w598, f=T4."j") -> (s? t:f=w602:T4)
            n405 = local write "part"(w602) -> ()
            "Step 2J" <- TRUE
          }
          frame "nothing" {
            n406 = local write "X Length"(0) -> ()
            n407 = local write "Y Length"(0) -> ()
          }
        }
      }
    }
    n408 = local read "y enetred"() -> (w71:dbl)
    n409 = local read "calc distance y"() -> (w70:dbl)
    n410 = local read "calc distanc x"() -> (w69:dbl)
    n411 = local read "x entered"() -> (w68:dbl)
    n412 = local read "stay"() -> (w65:dbl)
    n413 = local read "stay1"() -> (w64:dbl)
    n414 = formula code="if (Ylength==0)\nYerror=0;\n else  \nif(Ylength<0)\nYerror= Ylength+calculating_y_dis;\nelse\nYerror= Ylength-calculating_y_dis;\n\nif (stay==0)\nYerror=0;"("Ylength"=w71, "calculating_y_dis"=w70, "stay"=w65) -> ("Yerror"=→"error y":dbl)
    n415 = formula code="if (desired_xlength==0)\nXerror=0;\nelse\nif(desired_xlength>0)\nXerror=desired_xlength-actual_xLength;\nelse\nXerror=desired_xlength+actual_xLength;\n\nif (stay1==0)\nXerror=0;"("desired_xlength"=w68, "actual_xLength"=w69, "stay1"=w64) -> ("Xerror"=→"error x":dbl)
    n416 = local read "error y"() -> (w117:dbl)
    n417 = local read "error y"() -> (w116:dbl)
    n418 = local read "error x"() -> (w118:dbl)
    n419 = local read "error y"() -> (w132:dbl)
    n420 = local read "error y"() -> (w129:dbl)
    n421 = local read "error x"() -> (w125:dbl)
    n422 = local read "error x"() -> (w124:dbl)
    n423 = local read "error y"() -> (w133:dbl)
    n424 = local read "error x"() -> (w134:dbl)
    n425 = Less Than 0?(x=w117) -> (x < 0?=w115:bool)
    n426 = Less Than 0?(x=w118) -> (x < 0?=w114:bool)
    n427 = Greater Than 0?(x=w116) -> (x > 0?=w113:bool)
    n428 = Less Than 0?(x=w129) -> (x < 0?=w127:bool)
    n429 = Equal To 0?(x=w134) -> (x = 0?=w128:bool)
    n430 = Greater Than 0?(x=w132) -> (x > 0?=w131:bool)
    n431 = local read "error y"() -> (w110:dbl)
    n432 = local read "error x"() -> (w109:dbl)
    n433 = Greater Than 0?(x=w125) -> (x > 0?=w123:bool)
    n434 = Equal To 0?(x=w133) -> (x = 0?=w122:bool)
    n435 = Less Than 0?(x=w124) -> (x < 0?=w121:bool)
    n436 = And(x=w115, y=w114) -> (x .and. y?=w111:bool)
    n437 = And(x=w114, y=w113) -> (x .and. y?=w112:bool)
    n438 = And(x=w131, y=w128) -> (x .and. y?=w130:bool)
    n439 = And(x=w128, y=w127) -> (x .and. y?=w126:bool)
    n440 = local read "error y"() -> (w105:dbl)
    n441 = And(x=w123, y=w122) -> (x .and. y?=w120:bool)
    n442 = And(x=w122, y=w121) -> (x .and. y?=w119:bool)
    n443 = Greater Than 0?(x=w110) -> (x > 0?=w108:bool)
    n444 = Greater Than 0?(x=w109) -> (x > 0?=w106:bool)
    n445 = Less Than 0?(x=w105) -> (x < 0?=w104:bool)
    n446 = And(x=w108, y=w106) -> (x .and. y?=w107:bool)
    n447 = And(x=w106, y=w104) -> (x .and. y?=w103:bool)
    n448 = Select(t=1, s=w130, f=0) -> (s? t:f=w193:i32)
    n449 = Select(t=10, s=w119, f=0) -> (s? t:f=w191:i32)
    n450 = Select(t=2, s=w126, f=0) -> (s? t:f=w192:i32)
    n451 = Select(t=100, s=w107, f=0) -> (s? t:f=w189:i32)
    n452 = Select(t=200, s=w111, f=0) -> (s? t:f=w188:i32)
    n453 = Select(t=20, s=w120, f=0) -> (s? t:f=w190:i32)
    n454 = Select(t=1000, s=w112, f=0) -> (s? t:f=w187:i32)
    n455 = Select(t=2000, s=w103, f=0) -> (s? t:f=w173:i32)
    n456 = Add(x=w193, y=w192) -> (x+y=w186:i32)
    n457 = Add(x=w191, y=w190) -> (x+y=w185:i32)
    n458 = Add(x=w189, y=w188) -> (x+y=w184:i32)
    n459 = Add(x=w187, y=w173) -> (x+y=w172:i32)
    n460 = Add(x=w186, y=w185) -> (x+y=w183:i32)
    n461 = Add(x=w184, y=w172) -> (x+y=w171:i32)
    n462 = call-poly <vilib>:"DAQmx Read.vi"("task/channels in"=w224, "error in"=w222) -> ("task out"=w223:refnum<k21>, "data"=w155:bool, "error out"=w221:errorcluster)  [unwired: 11 in]
    "Top" <- w155
    n463 = call-poly <vilib>:"DAQmx Read.vi"("task/channels in"=w220, "error in"=w217) -> ("task out"=w214:refnum<k21>, "data"=w164:bool, "error out"=w211:errorcluster)  [unwired: 11 in]
    "Bottom" <- w164
    n464 = call-poly <vilib>:"DAQmx Read.vi"("task/channels in"=w219, "error in"=w216) -> ("task out"=w213:refnum<k21>, "data"=w163:bool, "error out"=w210:errorcluster)  [unwired: 11 in]
    "Right" <- w163
    n465 = call-poly <vilib>:"DAQmx Read.vi"("task/channels in"=w218, "error in"=w215) -> ("task out"=w212:refnum<k21>, "data"=w162:bool, "error out"=w209:errorcluster)  [unwired: 11 in]
    "Left" <- w162
    n466 = Add(x=w183, y=w171) -> (x+y=w102:i32)
    "direction selected" <- w102
    n467 = local read "check instruc"() -> (w77:bool)
    n468 = Multiply(x="Y Length", y=10) -> (x*y=w87:dbl)
    "y enetred" <- w87
    n469 = local read "Pulses M1"() -> (w144:dbl)
    n470 = Boolean To (0,1)(Boolean=w77) -> (0, 1=w76:i16)
    n471 = local read "Pulses M2"() -> (w148:dbl)
    n472 = Divide(x=w144, y=52.56) -> (x/y=→"p1 dis":dbl)
    n473 = feedback #1() -> (w84:dbl)  [unwired: 1 in]
    "calc distance y" <- w84
    n474 = formula code="Yerror=  (abs(Ylength)- abs(calculating_y_dis));\nif (Yerror<0.07)\nstay=0;\nif (stay==0)\nYerror=0;"("Ylength"=w87, "calculating_y_dis"=w84, "stay"=1, "circle"=w76) -> ("Yerror"=w136:dbl, "stay"=→"stay":i32)
    n475 = Divide(x=w148, y=52.56) -> (x/y=→"p1 dis 2":dbl)
    n476 = formula code="X=((PulseM1/52.56)+(PulseM2/52.56))/2.0;\nY=((PulseM1/52.56)+(PulseM2/52.56))/2.0;"("PulseM1"=w144, "PulseM2"=w148) -> ("X"=w51:dbl, "Y"=w52:dbl)
    "calc distanc x" <- w51
    n477 = feedback-in #1(w52) -> ()
    n478 = xnode "PID"("Error"=w136) -> ("Output"=w80:dbl)  [unwired: 2 in, 11 out]
    n479 = Multiply(x="X Length", y=10) -> (x*y=w90:dbl)
    "x entered" <- w90
    n480 = formula code="Xerror=(abs(desired_xlength)-abs(actual_xLength));\n\nif (Xerror<0.07)\nstay1 =0;\nif (stay1==0)\nXerror=0;"("actual_xLength"=w51, "desired_xlength"=w90, "stay1"=1) -> ("Xerror"=w135:dbl, "stay1"=→"stay1":i32)
    "error calced" <- w135
    n481 = case shown="10" w102 {
      tunnel: "motor 1" -> [w1286 w1289 w1292 w1299 w1303 w1307 w1313 w1319 w1325 w1330 w1337]
      tunnel: "motor 2" -> [w1283 w1291 w1294 w1297 w1302 w1305 w1311 w1317 w1323 w1331 w1336]
      tunnel: [w1282 w1291 w1293 w1296 w1302 w1304 w1310 w1316 w1322 w1328 w1335] -> w88
      tunnel: [w1285 w1288 w1292 w1298 w1303 w1306 w1312 w1318 w1324 w1329 w1334] -> w89
      frame 0, Default {
        n482 = Multiply(x=0, y=w1286) -> (x*y=w1285:dbl)
        n483 = Multiply(x=0, y=w1283) -> (x*y=w1282:dbl)
      }
      frame 1 {
        n484 = Multiply(x=-1, y=w1289) -> (x*y=w1288:dbl)
      }
      frame 2 {
        n485 = Multiply(x=-1.003, y=w1294) -> (x*y=w1293:dbl)
      }
      frame 10 {
        n486 = Multiply(x=-1, y=w1299) -> (x*y=w1298:dbl)
        n487 = Multiply(x=-1.1, y=w1297) -> (x*y=w1296:dbl)
      }
      frame 20 {
      }
      frame 100 {
        n488 = Multiply(x=0, y=w1307) -> (x*y=w1306:dbl)
        n489 = Multiply(x=1, y=w1305) -> (x*y=w1304:dbl)
      }
      frame 200 {
        n490 = Multiply(x=0, y=w1313) -> (x*y=w1312:dbl)
        n491 = Multiply(x=-1, y=w1311) -> (x*y=w1310:dbl)
      }
      frame 1000 {
        n492 = Multiply(x=-1, y=w1319) -> (x*y=w1318:dbl)
        n493 = Multiply(x=0, y=w1317) -> (x*y=w1316:dbl)
      }
      frame 2000 {
        n494 = Multiply(x=1, y=w1325) -> (x*y=w1324:dbl)
        n495 = Multiply(x=0, y=w1323) -> (x*y=w1322:dbl)
      }
      frame 4000 {
        n496 = Multiply(x=-1, y=w1330) -> (x*y=w1329:dbl)
        n497 = Multiply(x=0, y=w1331) -> (x*y=w1328:dbl)
      }
      frame 8000 {
        n498 = Multiply(x=-1, y=w1337) -> (x*y=w1334:dbl)
        n499 = Multiply(x=0, y=w1336) -> (x*y=w1335:dbl)
      }
    }
    n500 = Greater?(x=w80, y=-0.07) -> (0:w75:bool)
    n501 = Less?(x=w80, y=0.07) -> (x < y?=w74:bool)
    n502 = local read "Numeric"() -> (w138:dbl)
    n503 = And(x=w75, y=w74) -> (x .and. y?=w97:bool)
    "reached y" <- w97
    n504 = Multiply(x=0, y=w80) -> (x*y=w101:dbl)
    n505 = Select(t=w101, s=w97, f=w80) -> (s? t:f=→"calculating error y":dbl)
    n506 = Or(x=w164, y=w163) -> (x .or. y?=w207:bool)
    n507 = local read "Draw circle"() -> (w142:bool)
    n508 = And(x=w162, y=w155) -> (x .and. y?=w139:bool)
    n509 = local read "rectangle"() -> (w141:bool)
    n510 = Exclusive Or(1:w155, 2:w162) -> (0:w169:bool)
    n511 = Select(t=1, s=w162, f=0) -> (s? t:f=w154:i32)
    n512 = Select(t=2, s=w155, f=w154) -> (s? t:f=w159:i32)
    n513 = local read "check instruc"() -> (w83:bool)
    n514 = local read "Has encoders been reset?"() -> (w85:enum16{"don't reset", "reset"})
    n515 = xnode "PID 2"("Error"=w135) -> ("Output"=w79:dbl)  [unwired: 2 in, 11 out]
    n516 = Or(x=w142, y=w141) -> (x .or. y?=w82:bool)
    n517 = Select(t=1, s=w169, f=w138) -> (s? t:f=w168:dbl)
    n518 = Select(t=2, s=w139, f=w168) -> (s? t:f=w166:dbl)
    n519 = Or(x=w82, y=w83) -> (x .or. y?=w81:bool)
    n520 = Greater?(x=w79, y=-0.07) -> (0:w93:bool)
    "greater -1 x" <- w93
    n521 = Less?(x=w79, y=0.07) -> (x < y?=w94:bool)
    "less 1 x" <- w94
    n522 = call "Number To Enum.vim"("number"=w159, "enum type"=enum16{"Nothing", "Left", "Top"}."Nothing") -> ("number as enum"=w156:enum16{"Nothing", "Left", "Top"})
    n523 = case shown="True" "origin" {
      selector: "origin" -> [w1259 w1267]
      tunnel: [w1259 w1267] -> w170
      tunnel: w156 -> [_ w1260]
      frame False {
      }
      frame True {
        n524 = local read "Numeric"() -> (w1265:dbl)
        n525 = local read "Shape drawing steps"() -> (w1262:enum16{"corner", "1st switch", "reverse"})
        n526 = Equal?(x=w1265, y=2) -> (x = y?=w1264:bool)
        n527 = Select(t=enum16{"corner", "1st switch", "reverse"}."reverse", s=w1264, f=w1262) -> (s? t:f=w1261:enum16{"corner", "1st switch", "reverse"})
        n528 = case shown="\"1st switch\"" w1261 {
          tunnel: w1260 -> [_ w1271 _]
          frame "corner" {
            n529 = local write "Y Length"(50) -> ()
            n530 = local write "Has encoders been reset?"(enum16{"don't reset", "reset"}."don't reset") -> ()
            n531 = local write "X Length"(-50) -> ()
          }
          frame "1st switch" {
            n532 = case shown="\"Top\"" w1271 {
              frame "Nothing", Default {
                n533 = local write "Y Length"(0) -> ()
                n534 = local write "X Length"(0) -> ()
                n535 = local write "Numeric"(2) -> ()
              }
              frame "Left" {
                n536 = local write "X Length"(0) -> ()
                n537 = local write "Y Length"(50) -> ()
              }
              frame "Top" {
                n538 = local write "X Length"(-50) -> ()
                n539 = local write "Y Length"(0) -> ()
              }
            }
            n540 = local write "Has encoders been reset?"(enum16{"don't reset", "reset"}."don't reset") -> ()
          }
          frame "reverse" {
            n541 = local write "Has encoders been reset?"(enum16{"don't reset", "reset"}."reset") -> ()
            "Numeric" <- 2
          }
        }
      }
    }
    "In drawing mode" <- w170
    n542 = case shown="True" w81 {
      tunnel: w147 -> [w747 w752]
      tunnel: w146 -> [w748 w751]
      tunnel: [w745 w750] -> w145
      frame False {
        n543 = call-poly <vilib>:"DAQmx Read.vi"("task/channels in"=w747, "error in"=w748) -> ("data"=w746:dbl, "error out"=w745:errorcluster)  [unwired: 11 in, 1 out]
        n544 = local write "Pulses M1"(w746) -> ()
      }
      frame True {
        n545 = case shown="\"don't reset\", Default" "Has encoders been reset?" {
          tunnel: w752 -> [w756 w763]
          tunnel: w751 -> [w755 w762]
          tunnel: [w753 w764] -> w750
          frame "don't reset", Default {
            n546 = call-poly <vilib>:"DAQmx Read.vi"("task/channels in"=w756, "error in"=w755) -> ("data"=→"Pulses M1":dbl, "error out"=w753:errorcluster)  [unwired: 11 in, 1 out]
          }
          frame "reset" {
            n547 = call <vilib>:"DAQmx Stop Task.vi"("task/channels in"=w763, "error in"=w762) -> ("task out"=w761:refnum<k21>, "error out"=w760:errorcluster)  [unwired: 12 in]
            n548 = call <vilib>:"DAQmx Start Task.vi"("task/channels in"=w761, "error in"=w760) -> ("task out"=w759:refnum<k21>, "error out"=w758:errorcluster)  [unwired: 12 in]
            n549 = call-poly <vilib>:"DAQmx Read.vi"("task/channels in"=w759, "error in"=w758) -> ("data"=w757:dbl, "error out"=w764:errorcluster)  [unwired: 11 in, 1 out]
            n550 = local write "Pulses M1"(w757) -> ()
          }
        }
      }
    }
    n551 = case shown="True" w81 {
      tunnel: w143 -> [w736 w738]
      tunnel: w85 -> [_ w737]
      frame False {
        n552 = call-poly <vilib>:"DAQmx Read.vi"("task/channels in"=w736) -> ("data"=w735:dbl)  [unwired: 12 in, 2 out]
        n553 = local write "Pulses M2"(w735) -> ()
      }
      frame True {
        n554 = case shown="\"don't reset\", Default" w737 {
          tunnel: w738 -> [w740 w743]
          frame "don't reset", Default {
            n555 = call-poly <vilib>:"DAQmx Read.vi"("task/channels in"=w740) -> ("data"=→"Pulses M2":dbl)  [unwired: 12 in, 2 out]
          }
          frame "reset" {
            n556 = call <vilib>:"DAQmx Stop Task.vi"("task/channels in"=w743) -> ("task out"=w742:refnum<k21>)  [unwired: 13 in, 1 out]
            n557 = call <vilib>:"DAQmx Start Task.vi"("task/channels in"=w742) -> ("task out"=w744:refnum<k21>)  [unwired: 13 in, 1 out]
            n558 = call-poly <vilib>:"DAQmx Read.vi"("task/channels in"=w744) -> ("data"=w741:dbl)  [unwired: 12 in, 2 out]
            n559 = local write "Pulses M2"(w741) -> ()
          }
        }
      }
    }
    n560 = call "Number To Enum.vim"("number"=w166, "enum type"=enum16{"corner", "1st switch", "reverse"}."corner") -> ("number as enum"=→"Shape drawing steps":enum16{"corner", "1st switch", "reverse"})
    n561 = And(x=w93, y=w94) -> (x .and. y?=w96:bool)
    n562 = Multiply(x=0, y=w79) -> (x*y=w99:dbl)
    n563 = feedback-in #2(w96) -> ()
    n564 = feedback #2() -> (w95:bool)  [unwired: 1 in]
    "reached x" <- w95
    n565 = And(x=w97, y=w95) -> (x .and. y?=w153:bool)
    n566 = Or(x=w207, y=w153) -> (x .or. y?=w206:bool)
    n567 = Or(x=w206, y="Motor stop") -> (x .or. y?=w208:bool)
    n568 = Or(x=w208, y="stop") -> (x .or. y?=w228:bool)
    n569 = Select(t=0.0, s=w228, f=w88) -> (s? t:f=w225:dbl)
    n570 = call-poly <vilib>:"DAQmx Write.vi"("task/channels in"=w234, "data"=w225, "error in"=w231) -> ("task out"=w235:refnum<k21>, "error out"=w236:errorcluster)  [unwired: 10 in, 1 out]
    n571 = Select(t=0.0 ("s? t:f"), s=w228, f=w89) -> (s? t:f=w226:dbl)
    n572 = call-poly <vilib>:"DAQmx Write.vi"("task/channels in"=w240, "data"=w226, "error in"=w230) -> ("task out"=w239:refnum<k21>, "error out"=w238:errorcluster)  [unwired: 10 in, 1 out]
    n573 = call <vilib>:"DAQmx Wait Until Done.vi"("task/channels in"=w239, "error in"=w238) -> ("error out"=w237:errorcluster)  [unwired: 12 in, 1 out]
    n574 = call <vilib>:"DAQmx Wait Until Done.vi"("task/channels in"=w235, "error in"=w236) -> ("error out"=w233:errorcluster)  [unwired: 12 in, 1 out]
    n575 = Select(t=w99, s=w95, f=w79) -> (s? t:f=→"calculating error x":dbl)
  }
  n576 = invoke on="motor 1" class="Slide (strict)" method="Reinit To Default"() -> ()  [unwired: 3 in, 3 out]
  n577 = invoke on="Numeric" class="DigNum (strict)" method="Reinit To Default"() -> ()  [unwired: 3 in, 3 out]
  n578 = invoke on="No of Points" class="DigNum (strict)" method="Reinit To Default"() -> ()  [unwired: 3 in, 3 out]
  n579 = invoke on="Shape drawing steps" class="Enum (strict)" method="Reinit To Default"() -> ()  [unwired: 3 in, 3 out]
  n580 = invoke on="part" class="Enum (strict)" method="Reinit To Default"() -> ()  [unwired: 3 in, 3 out]
  n581 = invoke on="stage circle" class="Enum (strict)" method="Reinit To Default"() -> ()  [unwired: 3 in, 3 out]
  n582 = invoke on="array Y length 2" class="DigNum (strict)" method="Reinit To Default"() -> ()  [unwired: 3 in, 3 out]
  n583 = invoke on="c" class="Bool (strict)" method="Reinit To Default"() -> ()  [unwired: 3 in, 3 out]
  n584 = invoke on="at 2f" class="Bool (strict)" method="Reinit To Default"() -> ()  [unwired: 3 in, 3 out]
  n585 = invoke on="reached x" class="Bool (strict)" method="Reinit To Default"() -> ()  [unwired: 3 in, 3 out]
  n586 = invoke on="array x Length 2" class="DigNum (strict)" method="Reinit To Default"() -> ()  [unwired: 3 in, 3 out]
  n587 = invoke on="Step 2D" class="Bool (strict)" method="Reinit To Default"() -> ()  [unwired: 3 in, 3 out]
  n588 = invoke on="Step 2H" class="Bool (strict)" method="Reinit To Default"() -> ()  [unwired: 3 in, 3 out]
  n589 = invoke on="Point circle is drawing" class="DigNum (strict)" method="Reinit To Default"() -> ()  [unwired: 3 in, 3 out]
  n590 = invoke on="reached y" class="Bool (strict)" method="Reinit To Default"() -> ()  [unwired: 3 in, 3 out]
  n591 = invoke on="Step 2E" class="Bool (strict)" method="Reinit To Default"() -> ()  [unwired: 3 in, 3 out]
  n592 = invoke on="Step 2J" class="Bool (strict)" method="Reinit To Default"() -> ()  [unwired: 3 in, 3 out]
  n593 = invoke on="previous index" class="DigNum (strict)" method="Reinit To Default"() -> ()  [unwired: 3 in, 3 out]
  n594 = invoke on="stage rectangle" class="Enum (strict)" method="Reinit To Default"() -> ()  [unwired: 3 in, 3 out]
  n595 = call <vilib>:"Simple Error Handler.vi"("error source (\" \")"="you messed up" ("error source (\" \")"), "error in (no error)"=w48) -> ()  [unwired: 3 in, 5 out]
  n596 = call <vilib>:"Simple Error Handler.vi"("error source (\" \")"="you messed up" ("error source (\" \")"), "error in (no error)"=w45) -> ()  [unwired: 3 in, 5 out]
  n597 = call <vilib>:"DAQmx Clear Task.vi"("task in"=w27, "error in"=w25) -> ()  [unwired: 13 in, 1 out]
  n598 = call <vilib>:"DAQmx Clear Task.vi"("task in"=w17, "error in"=w14) -> ()  [unwired: 13 in, 1 out]
  n599 = call <vilib>:"DAQmx Clear Task.vi"("task in"=w18, "error in"=w15) -> ("error out"=w12:errorcluster)  [unwired: 13 in]
  n600 = call <vilib>:"DAQmx Clear Task.vi"("task in"=w16, "error in"=w13) -> ()  [unwired: 13 in, 1 out]
  n601 = call <vilib>:"Simple Error Handler.vi"("error in (no error)"=w12) -> ()  [unwired: 4 in, 5 out]
  n602 = call <vilib>:"Simple Error Handler.vi"("error source (\" \")"="you messed up" ("error source (\" \")"), "error in (no error)"=w10) -> ()  [unwired: 3 in, 5 out]
